vi "Non Callback Test.vi"() -> ()   [LabVIEW 2011]
uses:
  <vilib>/vision/Image Controls.llb/IMAQ Image.ctl
  <vilib>/Platform/TimedLoop/XDataNode/timing_clust.ctl
  <vilib>/Platform/TimedLoop/XDataNode/nitl_modes.ctl
  <vilib>/Platform/TimedLoop/XDataNode/wakeup.ctl
  C:/Users/Behavior Room/Desktop/Kinect Mouse/DepthSense/FunctionPointerProxy/FunctionPointerProxy/bin/Release/FunctionPointerProxy.dll
  FunctionPointerProxy/FunctionPointerProxy/bin/Release/FunctionPointerProxy.dll
  DepthSense Global Status.vi
  <vilib>/Platform/TimedLoop/XDataNode/XDataNode.xnode
  <userlib>/libOptrima-2-3/libOptrima-2-3.lvlib
  <vilib>/Platform/TimedLoop/XDataNode/XDNodeRunTimeDep.lvlib
  Program Files (x86)/SoftKinetic/OptrimaSDK/lib/libOptrima-2-3.dll
panel:
  out "Image":T1(plugin-control)
  out "Frame ID":i32
  in  "DepthSense Indicator":T2={"Camera Version"="", "Image Height"=0, "Image Width"=0, "Minimum Framerate"=0, "Maximum Framerate"=0, "Framerate"=25, "Close Mode"=FALSE, "Denoising"=FALSE, "Leakage Algorithm"=FALSE, "Anti-Aliasing"=FALSE, "Camera Status"=-2, "API Version"="", "Light Intensity"=100, "Confidence Threshold"=100, "Range"=0.0}
  in  "stop":bool
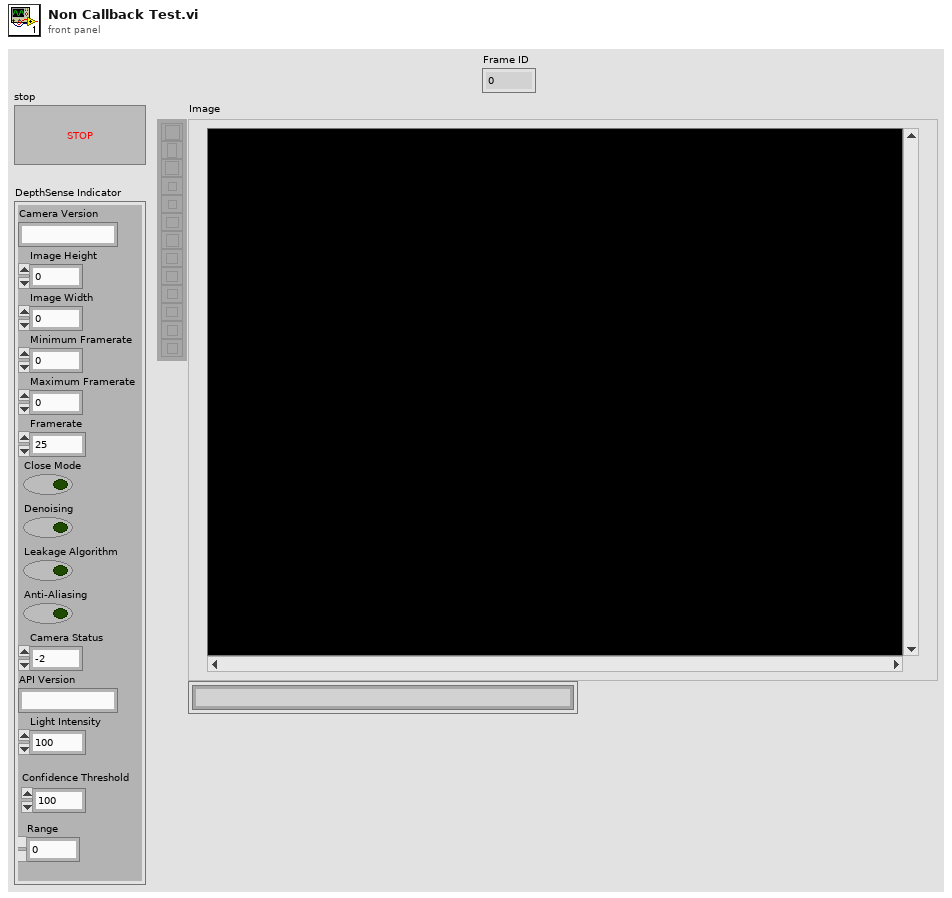
[diagram p1: front panel]
types:
  T1 = typedef "IMAQ Image.ctl" = refnum<image>
  T2 = cluster{"Camera Version":string, "Image Height":i32, "Image Width":i32, "Minimum Framerate":i32, "Maximum Framerate":i32, "Framerate":i32, "Close Mode":bool, "Denoising":bool, "Leakage Algorithm":bool, "Anti-Aliasing":bool, "Camera Status":i32, "API Version":string, "Light Intensity":i32, "Confidence Threshold":u16, "Range":dbl}
  T3 = cluster{"Camera Version":string, "Image Height":i32, "Image Width":i32, "Minimum Framerate":i32, "Maximum Framerate":i32, "Framerate":i32, "Close Mode":bool, "Denoising":bool, "Leakage Algorithm":bool, "Anti-Aliasing":bool, "Camera Status":i32, "API Version":string, "Light Intensity":i32, "Confidence Threshold":u16, "Range":sgl}
  T4 = typedef "t_CallbackReferences.ctl" = cluster{"LV event callback ":refnum<k27>, "Proxy instance":refnum<k24>, "(*f)(...)":i32}
  T5 = typedef "XDNodeRunTimeDep.lvlib/timing_clust.ctl" = cluster{"Expected End [f-1]":u64, "Actual End [f-1]":u64, "Finished Late? [f-1]":bool, "Expected End [i-1]":u64, "Actual End [i-1]":u64, "Finished Late? [i-1]":bool, "Expected Start [i]":u64, "Actual Start [i]":u64, "Expected Start [f]":u64, "Actual Start [f]":u64, "Source Name":string, "Structure Name":string, "Period":i64, "Deadline":i64, "Offset":i64, "Start":i64, "Priority":i32, "Timeout":i32, "Mode":T6, "Wakeup Reason":T7, "Error":errorcluster, "Source Type":string, "Secondary Source Type":string, "Global End Time":u64, "Global Start Time":u64, "Frame Duration":u64, "Iteration Duration":u64, "Assigned CPU":i32, "I/O Scan Engine Mode":u32}
  T6 = typedef "XDNodeRunTimeDep.lvlib/nitl_modes.ctl" = enum32{"No Change", "Process missed periods, maintain original phase", "Discard missed periods, maintain original phase", "Process missed periods, ignore original phase", "Discard missed periods, ignore original phase"}
  T7 = typedef "XDNodeRunTimeDep.lvlib/wakeup.ctl" = enum32{"Normal", "Aborted", "Asynchronous wakeup", "Timing source error", "Timed loop error", "Timeout"}
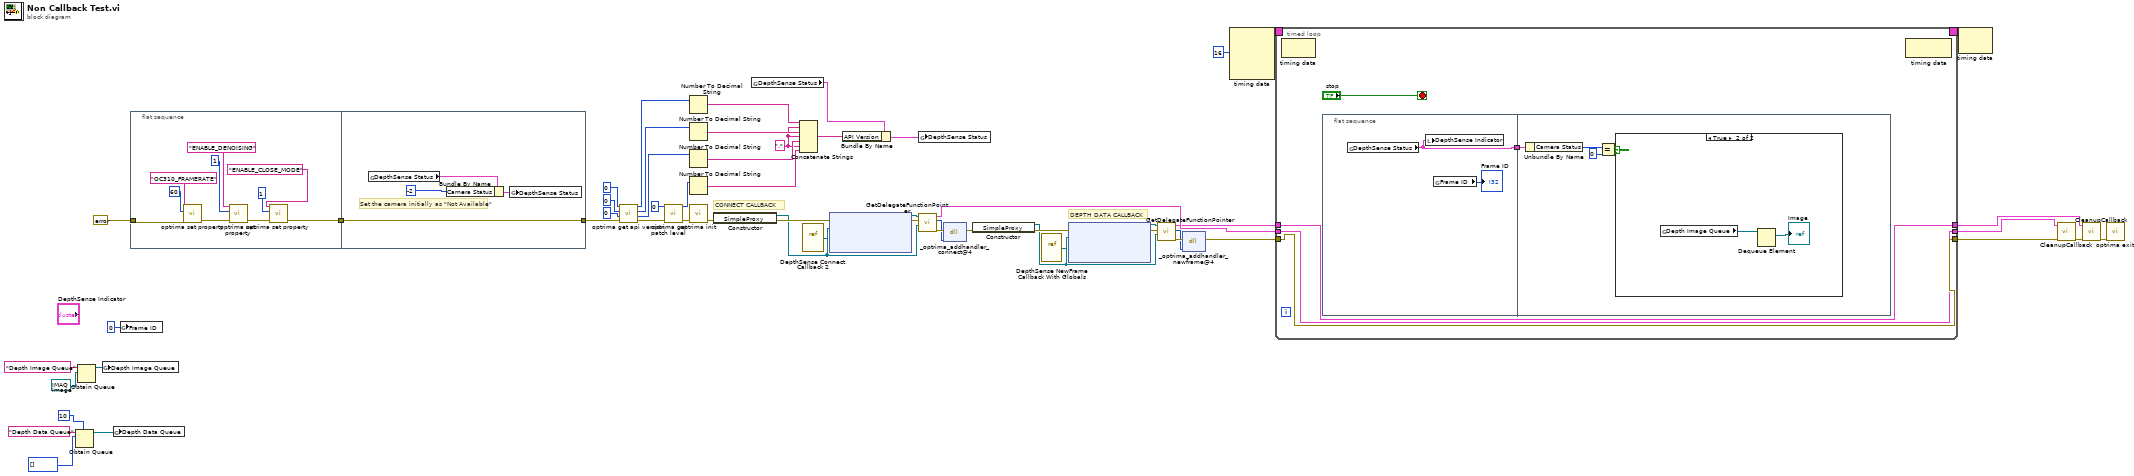
[diagram p0: block diagram]
diagram:
  w43 = "."
  # "DEPTH DATA CALLBACK"
  # "CONNECT CALLBACK"
  n1 = Obtain Queue(max queue size (-1, unlimited)=10, name (unnamed)="Depth Data Queue", element data type=i16[] [] ("output array")) -> (queue out=w1:refnum<queue>)  [unwired: 2 in, 2 out]
  n2 = Obtain Queue(name (unnamed)="Depth Image Queue", element data type=T1 refnum ("New Image")) -> (queue out=w32:refnum<queue>)  [unwired: 3 in, 2 out]
  n3 = global write "DepthSense Global Status.vi" "Depth Image Queue"(w32) -> ()
  n4 = global write "DepthSense Global Status.vi" "Depth Data Queue"(w1) -> ()
  n5 = global write "DepthSense Global Status.vi" "Frame ID"(0 ("Frame ID")) -> ()
  n6 = flat-sequence {
    tunnel: errorcluster {"status"=FALSE, "code"=0, "source"=""} ("error in (no error)") -> [w57]
    tunnel: [w60] -> w9
    tunnel: [w68] -> w13
    tunnel: w9 -> [w68]
    frame #0 {
      n7 = call <userlib>:"optrima set property.vi"("error in (no error)"=w57, "value"=u32 60, "name"="OC310_FRAMERATE") -> ("error out"=w62:errorcluster)  [unwired: 7 in, 1 out]
      n8 = call <userlib>:"optrima set property.vi"("error in (no error)"=w62, "value"=u32 1, "name"="ENABLE_DENOISING") -> ("error out"=w61:errorcluster)  [unwired: 7 in, 1 out]
      n9 = call <userlib>:"optrima set property.vi"("error in (no error)"=w61, "value"=u32 1, "name"="ENABLE_CLOSE_MODE") -> ("error out"=w60:errorcluster)  [unwired: 7 in, 1 out]
    }
    frame #1 {
      # "Set the camera initially as \"Not Available\""
      n10 = global read "DepthSense Global Status.vi" "DepthSense Status"() -> (w67:T3)
      n11 = Bundle By Name(cluster=w67, "Camera Status"=-2) -> (w70:T3)
      n12 = global write "DepthSense Global Status.vi" "DepthSense Status"(w70) -> ()
    }
  }
  n13 = call <userlib>:"optrima get api version.vi"("error in (no error)"=w13, "minor"=u32 0, "major"=u32 0, "release"=u32 0) -> ("error out"=w56:errorcluster, "minor out"=w53:u32, "major out"=w54:u32, "release out"=w55:u32)  [unwired: 4 in]
  n14 = call <userlib>:"optrima get patch level.vi"("error in (no error)"=w56, "patch"=u32 0) -> ("error out"=w12:errorcluster, "patch out"=w52:u32)  [unwired: 8 in]
  n15 = Number To Decimal String(number=w55) -> (decimal integer string=w51:string)  [unwired: 1 in]
  n16 = Number To Decimal String(number=w54) -> (decimal integer string=w46:string)  [unwired: 1 in]
  n17 = Number To Decimal String(number=w53) -> (decimal integer string=w45:string)  [unwired: 1 in]
  n18 = Number To Decimal String(number=w52) -> (decimal integer string=w44:string)  [unwired: 1 in]
  n19 = call <userlib>:"optrima init.vi"("error in (no error)"=w12) -> ("error out"=w11:errorcluster)  [unwired: 10 in]
  n20 = constructor class="SimpleProxy"(error in=w11) -> (reference out=w39:refnum<k24>, error out=w42:errorcluster)  [unwired: 2 in, 1 out]
  n21 = global read "DepthSense Global Status.vi" "DepthSense Status"() -> (w15:T3)
  n22 = Concatenate Strings(w51, w43, w46, w43, w45, w43, w44) -> (w35:string)
  n23 = vi-ref "DepthSense Connect Callback 2.vi"() -> ("vi reference"=w31:refnum<vi>)
  n24 = node(w42, w39, w31) -> (w41:refnum<k27>, w40:errorcluster)  [unwired: 2 in]
  n25 = Bundle By Name(cluster=w15, "API Version"=w35) -> (w16:T3)
  n26 = global write "DepthSense Global Status.vi" "DepthSense Status"(w16) -> ()
  n27 = call "GetDelegateFunctionPointer.vi"("target class"=w39, "error in (no error)"=w40, "event callback refnum"=w41) -> ("error out"=w38:errorcluster, "(*f)(...)"=w37:i32, "References"=w36:T4)  [unwired: 6 in]
  n28 = dll-call lib="C:/Program Files (x86)/SoftKinetic/OptrimaSDK/lib/libOptrima-2-3.dll" fn="_optrima_addhandler_connect@4"(error in=w38, "handlerfunc"=w37) -> (error out=w21:errorcluster)  [unwired: 4 in, 1 out]
  n29 = constructor class="SimpleProxy"(error in=w21) -> (reference out=w29:refnum<k24>, error out=w30:errorcluster)  [unwired: 2 in, 1 out]
  n30 = vi-ref "DepthSense NewFrame Callback With Globals.vi"() -> ("vi reference"=w24:refnum<vi>)
  n31 = node(w30, w29, w24) -> (w27:refnum<k27>, w28:errorcluster)  [unwired: 2 in]
  n32 = call "GetDelegateFunctionPointer.vi"("target class"=w29, "error in (no error)"=w28, "event callback refnum"=w27) -> ("error out"=w26:errorcluster, "(*f)(...)"=w25:i32, "References"=w23:T4)  [unwired: 6 in]
  n33 = dll-call lib="C:/Program Files (x86)/SoftKinetic/OptrimaSDK/lib/libOptrima-2-3.dll" fn="_optrima_addhandler_newframe@4"(error in=w26, "handlerfunc"=w25) -> (error out=w22:errorcluster)  [unwired: 4 in, 1 out]
  n34 = node-c288(i64 16 ("Period")) -> (w4:T5)  [unwired: 3 in]
  n35 = timed-loop {
    tunnel: [w75] -> w5
    tunnel: w22 -> [w75]
    tunnel: [w74] -> w18
    tunnel: w36 -> [w74]
    tunnel: w23 -> [w73]
    tunnel: [w73] -> w17
    timing: w4 -> [_]
    timing-out: [_] -> w3
    stop <- "stop" stop-if-true
    n36 = node-c288() -> ()  [unwired: 1 in, 1 out]
    n37 = flat-sequence {
      tunnel: [w79] -> w72
      tunnel: w72 -> [w80]
      frame #0 {
        n38 = global read "DepthSense Global Status.vi" "DepthSense Status"() -> (w79:T3)
        n39 = local write "DepthSense Indicator"(w79) -> ()
        n40 = global read "DepthSense Global Status.vi" "Frame ID"() -> (→"Frame ID":i32)
      }
      frame #1 {
        n41 = Unbundle By Name(w80) -> ("Camera Status"=w82:i32)
        n42 = Equal?(x=w82, y=0) -> (x = y?=w83:bool)
        n43 = case shown="True" w83 {
          frame False {
          }
          frame True {
            n44 = global read "DepthSense Global Status.vi" "Depth Image Queue"() -> (w85:refnum<queue>)
            n45 = Dequeue Element(queue=w85) -> (element=→"Image":T1)  [unwired: 2 in, 3 out]
          }
        }
      }
    }
    n46 = node-c288() -> ()  [unwired: 1 in, 1 out]
  }
  n47 = node-c288(w3) -> ()  [unwired: 1 out]
  n48 = call "CleanupCallback.vi"("error in (no error)"=w5, "References"=w18) -> ("error out"=w19:errorcluster)  [unwired: 9 in]
  n49 = call "CleanupCallback.vi"("error in (no error)"=w19, "References"=w17) -> ("error out"=w20:errorcluster)  [unwired: 9 in]
  n50 = call <userlib>:"optrima exit.vi"("error in (no error)"=w20) -> ()  [unwired: 10 in, 1 out]
